vi "DriverStationSendData.vi"   [LabVIEW 2020]
doc: "This VI continously sends data from the robot to the FRC 4265 Dashboard, the joysticks, and the FIRST Driver Station. Data are only sent to the network tables when values change. Detailed sensor data are only sent when the user is currently viewing the Tune tab on the FRC 4265 Dashboard."
uses:
  GlobalDriverStationData.vi
  <vilib>/Rock Robotics/Network Tables/NT Write String Array.vi
  GlobalAutonomous.vi
  GlobalPoseAndTargeting.vi
  GlobalMiscellaneous.vi
  89115614-314f-44eb-b4c5-fafba5d31cd4.vi
  d5b4d43d-cd94-4278-ad04-5030dc28ac17.vi
  9f98788f-6f1b-4a83-a100-7d872b9f460c.vi
  47e8091e-0604-4560-b6ee-932fcc40f94c.vi
  d2dc3f3f-39b5-4c17-a933-05bbedc8d5d9.vi
  36759aca-d9c6-44a3-918a-9a0e895c718f.vi
  0620df73-5841-450f-a219-dd10bb38cbc0.vi
  fb087c59-fbb1-4979-ba7d-d29f083bcd8a.vi
  5739ca73-a30d-4c92-9c50-72d6edc45fc4.vi
  811948b9-57e2-4f47-a6f6-f2932d14082f.vi
  040c557e-2b24-4d13-8fef-d98c711cf45f.vi
  5dc304d7-e71b-4cd2-8d9d-954937278b50.vi
  296afef1-bc02-48ee-92b6-09523bb21575.vi
  5ccc8aa6-325d-4660-b060-52e30b1d582a.vi
  52d993e2-6fbc-4ee4-b085-b3f80a4c3067.vi
  63edfc8b-2713-4fb9-bbf0-712b13f7ed91.vi
  c0b3d222-824d-4eea-b194-4551ccfede72.vi
  cbbdf295-aa1d-4db8-8566-cac5820e4458.vi
  26471c2c-aca7-4047-a7cd-e40da11d04c1.vi
  a2a431f6-075f-4920-bddd-4a0a2690fbc3.vi
  d5b53c9f-0752-48c4-83e9-94c6e20357af.vi
  5e95d400-1295-40c5-af46-ec5444c3a2ff.vi
  20dd8ad3-6bbc-4cac-b559-7f798e2b6680.vi
  7b6a1411-5027-49fa-871d-ec9f81e31f95.vi
  c10cd8a7-bdb7-4c92-ac5c-00af4ab7dc85.vi
  07cec073-88f4-4f05-94a3-d05e12405c4e.vi
  948ebb5e-1fee-45f5-b788-843df8d92f11.vi
  0c9c2ce5-4f8f-4d2f-a61f-dde9fdddd21a.vi
  6883bb39-9618-44d1-87fc-0a8820399f5c.vi
  <vilib>/Rock Robotics/Network Tables/NT Write String.vi
  <vilib>/Rock Robotics/Network Tables/NT Write Number.vi
  90b8ffb3-02b0-4f37-8578-c415475fcf1f.vi
  fa7611ee-6daf-4341-84ec-bae2216748b8.vi
  94826c24-d30e-4eee-b4d4-6d626a9b9fe7.vi
  ce82ba1c-dcc2-498f-8d23-146b12230de2.vi
  e617f737-58a4-4889-9924-01a8da667f92.vi
  c227876e-c49d-4561-a8c1-0ac62d9f5df0.vi
  44842b00-b9c8-4b1f-a6e0-fc22f00ef89a.vi
  a9076398-35a2-42a7-b542-3dd64d126b59.vi
  GlobalDrivebase.vi
  0776bb0e-5b58-4af6-957d-bc8a00d122f2.vi
  <vilib>/Rock Robotics/WPI/DriverStation/WPI_DriverStationAllianceInfo.ctl
  <vilib>/Rock Robotics/Network Tables/NT Write Boolean.vi
  e0f98f21-d526-4ef5-b75c-6f3c78a33603.vi
  09cab74e-98ba-4de8-92cd-b77291f0cae9.vi
  bf36f1cc-a3b1-4189-9382-aff2debcdd91.vi
  9b798e4d-9237-4864-9935-e997a6382231.vi
  d8771982-752a-4faa-9266-2bef2163cf3a.vi
  12ad7fc7-8c22-4204-99a5-6d293ce0fad5.vi
  26bfd72d-5ff1-456c-8357-2895bcab42df.vi
  770be32f-1451-480f-be59-c95d907125ff.vi
  <vilib>/Rock Robotics/Network Tables/NT Write Float Array.vi
  8b25c428-5d86-4327-8799-14b0f475aaa3.vi
types:
  T1 = typedef "WPI_DriverStationAllianceInfo.ctl" = enum16{"Red", "Blue", "Invalid"}
  T2 = enum16{"Low Gear", "High Gear", "Transiting", "Unknown", "Force Low Gear"}
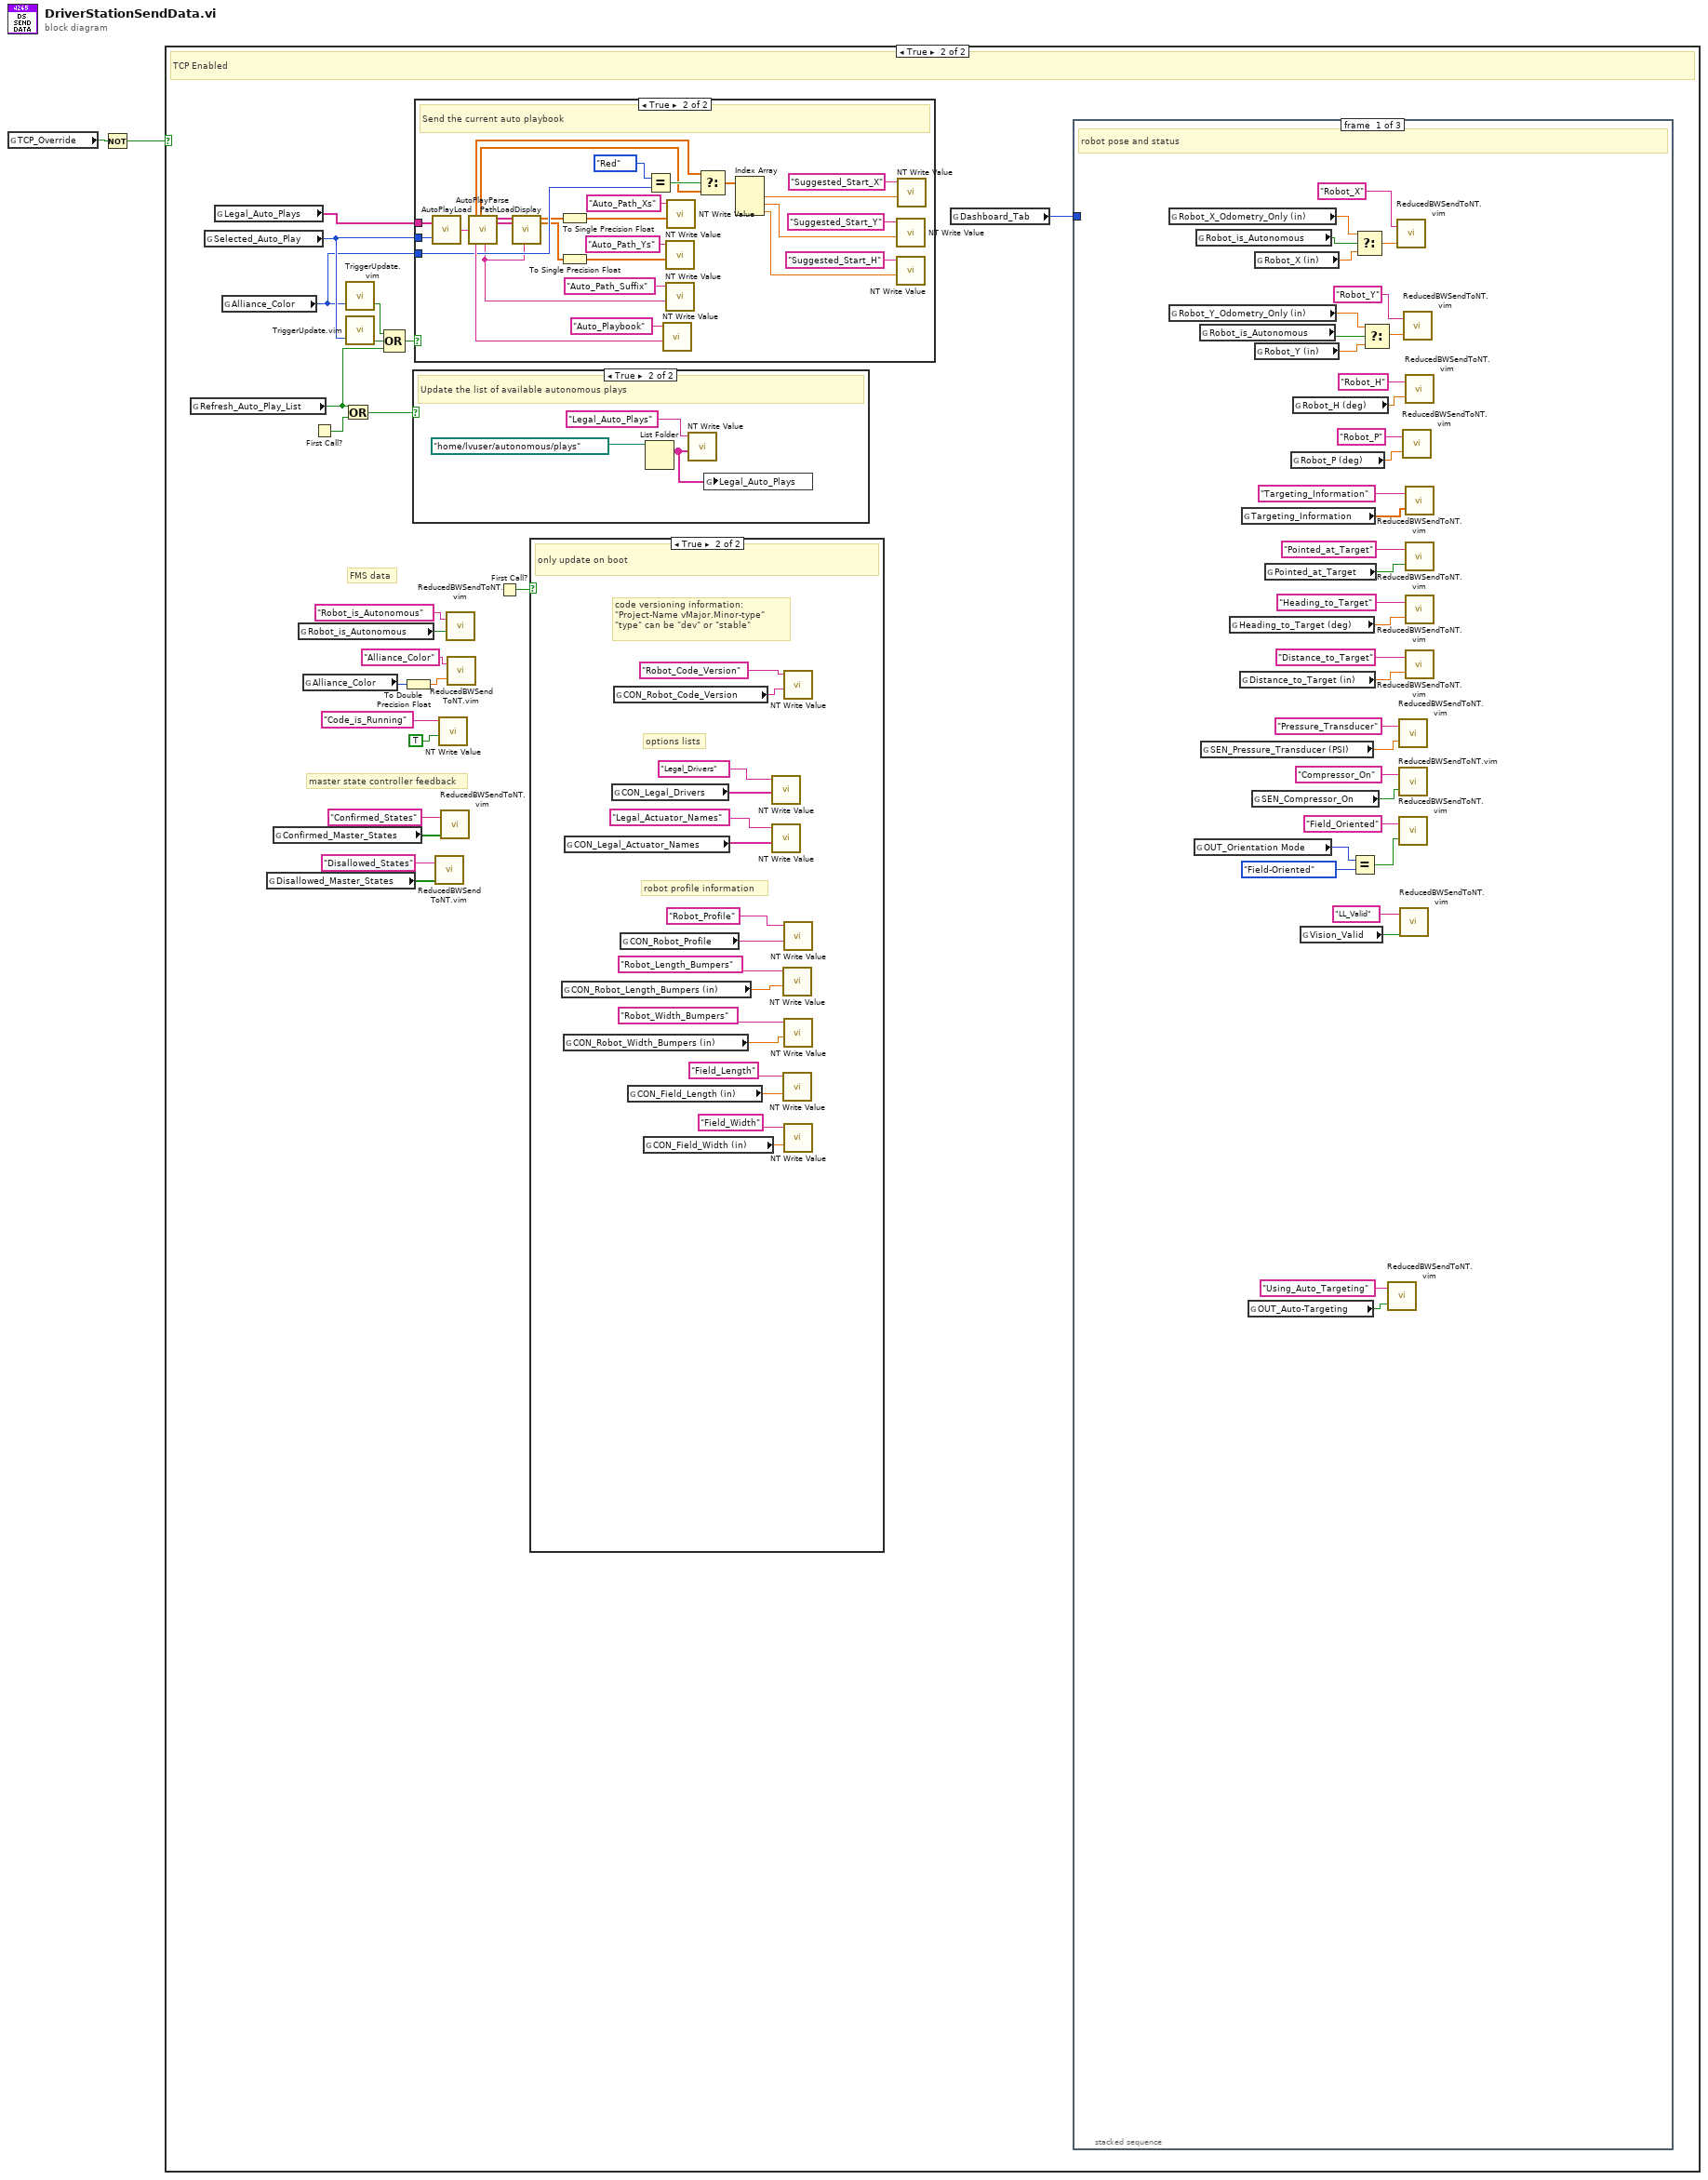
[diagram p0: block diagram]
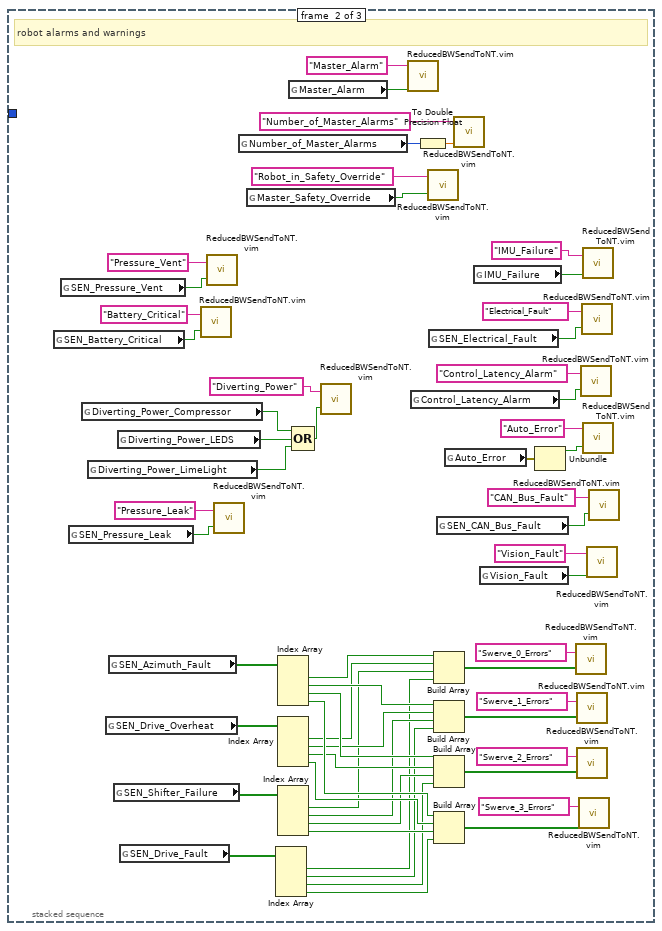
[diagram p3: hidden frame]
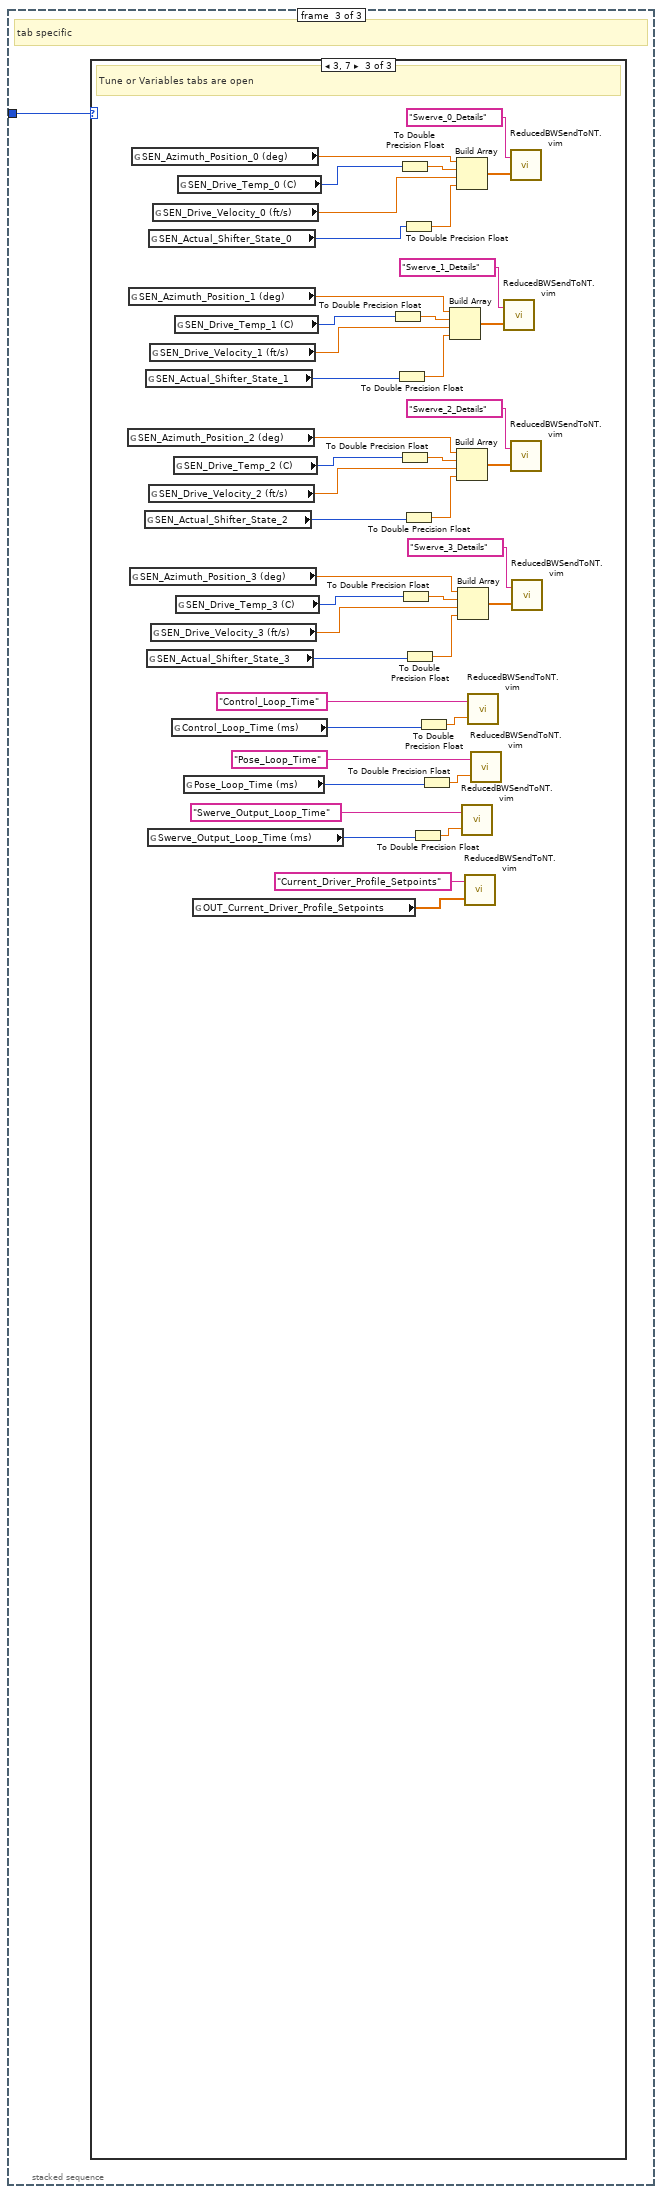
[diagram p4: hidden frame]
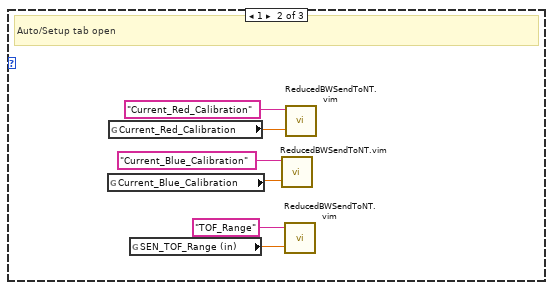
[diagram p6: hidden frame]
diagram:
  n1 = global read "GlobalDriverStationData.vi" "TCP_Override"() -> (w2:bool)
  n2 = Not(x=w2) -> (.not. x?=w1:bool)
  n3 = case shown="True" w1 {
    frame False {
      # "TCP Disabled"
    }
    frame True {
      # "FMS data"
      # "master state controller feedback"
      # "TCP Enabled"
      n4 = global read "GlobalDriverStationData.vi" "Refresh_Auto_Play_List"() -> (w20:bool)
      n5 = global read "GlobalDriverStationData.vi" "Selected_Auto_Play"() -> (w7:u16)
      n6 = global read "GlobalAutonomous.vi" "Legal_Auto_Plays"() -> (w8:string[])
      n7 = global read "GlobalDriverStationData.vi" "Alliance_Color"() -> (w5:T1)
      n8 = global read "GlobalMiscellaneous.vi" "Disallowed_Master_States"() -> (w10:bool[])
      n9 = global read "GlobalMiscellaneous.vi" "Confirmed_Master_States"() -> (w12:bool[])
      n10 = global read "GlobalDriverStationData.vi" "Robot_is_Autonomous"() -> (w16:bool)
      n11 = global read "GlobalDriverStationData.vi" "Alliance_Color"() -> (w18:T1)
      n12 = First Call?() -> (First Call?: T/F=w24:bool)
      n13 = Or(x=w20, y=w24) -> (x .or. y?=w23:bool)
      n14 = call "TriggerUpdate.vim"("Trigger"=w5) -> ("Update"=w6:bool)  [unwired: 2 in]
      n15 = call "TriggerUpdate.vim"("Trigger"=w7) -> ("Update"=w22:bool)  [unwired: 2 in]
      n16 = Compound Arithmetic op=OR(w6, w22, w20) -> (w21:bool)
      n17 = To Double Precision Float(number=w18) -> (double precision float=w14:dbl)
      n18 = case shown="True" w23 {
        frame False {
        }
        frame True {
          # "Update the list of available autonomous plays"
          n19 = List Folder(path=path "/home/lvuser/autonomous/plays") -> (filenames=w211:string[])  [unwired: 3 in, 3 out]
          n20 = call-poly <vilib>:"NT Write Value.vi"("value"=w211, "name"="Legal_Auto_Plays" ("Name")) -> ()  [unwired: 9 in, 1 out]
          n21 = global write "GlobalAutonomous.vi" "Legal_Auto_Plays"(w211) -> ()
        }
      }
      n22 = case shown="True" w21 {
        tunnel: w7 -> [_ w208]
        tunnel: w8 -> [_ w207]
        tunnel: w5 -> [_ w203]
        frame False {
        }
        frame True {
          # "Send the current auto playbook"
          n23 = call "AutoPlayLoad.vi"("Selected Auto Play"=w208, "Available Auto Plays"=w207) -> ("Loaded Auto Play"=w209:string)
          n24 = call "AutoPlayParse.vi"("Loaded Auto Play"=w209) -> ("Suggested Start Red"=w201:dbl[], "Full Auto Play Text"=w206:string, "Suggested Start Blue"=w200:dbl[], "Autonomous Path Suffix"=w190:string, "Drive Command Strings"=w192:string[], "Drive Parameter Strings"=w191:string[])  [unwired: 10 in, 3 out]
          n25 = call "PathLoadDisplay.vi"("Drive Command Strings"=w192, "Drive Parameter Strings"=w191, "Autonomous Path Suffix"=w190) -> ("Path X Coordinates (in)"=w188:dbl[], "Path Y Coordinates (in)"=w186:dbl[])  [unwired: 15 in]
          n26 = To Single Precision Float(number=w188) -> (single precision float=w185:sgl[])
          n27 = To Single Precision Float(number=w186) -> (single precision float=w184:sgl[])
          n28 = Equal?(x=WPI_DriverStationAllianceInfo."Red", y=w203) -> (x = y?=w204:bool)
          n29 = call-poly <vilib>:"NT Write Value.vi"("value"=w206, "name"="Auto_Playbook" ("Name")) -> ()  [unwired: 9 in, 1 out]
          n30 = call-poly <vilib>:"NT Write Value.vi"("value"=w184, "name"="Auto_Path_Ys" ("Name")) -> ()  [unwired: 9 in, 1 out]
          n31 = call-poly <vilib>:"NT Write Value.vi"("value"=w190, "name"="Auto_Path_Suffix" ("Name")) -> ()  [unwired: 9 in, 1 out]
          n32 = call-poly <vilib>:"NT Write Value.vi"("value"=w185, "name"="Auto_Path_Xs" ("Name")) -> ()  [unwired: 9 in, 1 out]
          n33 = Select(t=w201, s=w204, f=w200) -> (s? t:f=w199:dbl[])
          n34 = Index Array(array=w199) -> (element #1=w195:dbl, element #2=w194:dbl, element #3=w193:dbl)  [unwired: 3 in]
          n35 = call-poly <vilib>:"NT Write Value.vi"("value"=w194, "name"="Suggested_Start_Y" ("Name")) -> ()  [unwired: 9 in, 1 out]
          n36 = call-poly <vilib>:"NT Write Value.vi"("value"=w193, "name"="Suggested_Start_H" ("Name")) -> ()  [unwired: 9 in, 1 out]
          n37 = call-poly <vilib>:"NT Write Value.vi"("value"=w195, "name"="Suggested_Start_X" ("Name")) -> ()  [unwired: 9 in, 1 out]
        }
      }
      n38 = call "ReducedBWSendToNT.vim"("Value In"=w10, "NT Name"="Disallowed_States" ("Name")) -> ()  [unwired: 1 out]
      n39 = call-poly <vilib>:"NT Write Value.vi"("value"=TRUE, "name"="Code_is_Running" ("NT Name")) -> ()  [unwired: 9 in, 1 out]
      n40 = call "ReducedBWSendToNT.vim"("Value In"=w12, "NT Name"="Confirmed_States" ("Name")) -> ()  [unwired: 1 out]
      n41 = call "ReducedBWSendToNT.vim"("Value In"=w16, "NT Name"="Robot_is_Autonomous") -> ()  [unwired: 1 out]
      n42 = call "ReducedBWSendToNT.vim"("Value In"=w14, "NT Name"="Alliance_Color") -> ()  [unwired: 1 out]
      n43 = First Call?() -> (First Call?: T/F=w19:bool)
      n44 = case shown="True" w19 {
        frame False {
        }
        frame True {
          # "robot profile information"
          # "options lists"
          # "code versioning information:\n\"Project-Name vMajor.Minor-type\"\n\"type\" can be \"dev\" or \"stable\""
          # "only update on boot"
          n45 = global read "GlobalDrivebase.vi" "CON_Robot_Length_Bumpers (in)"() -> (w177:dbl)
          n46 = global read "GlobalDrivebase.vi" "CON_Robot_Width_Bumpers (in)"() -> (w176:dbl)
          n47 = global read "GlobalMiscellaneous.vi" "CON_Legal_Actuator_Names"() -> (w174:string[])
          n48 = global read "GlobalDrivebase.vi" "CON_Legal_Drivers"() -> (w175:string[])
          n49 = global read "GlobalMiscellaneous.vi" "CON_Robot_Code_Version"() -> (w172:string)
          n50 = global read "GlobalMiscellaneous.vi" "CON_Robot_Profile"() -> (w173:string)
          n51 = global read "GlobalPoseAndTargeting.vi" "CON_Field_Length (in)"() -> (w171:dbl)
          n52 = global read "GlobalPoseAndTargeting.vi" "CON_Field_Width (in)"() -> (w168:dbl)
          n53 = call-poly <vilib>:"NT Write Value.vi"("value"=w175, "name"="Legal_Drivers" ("Name")) -> ()  [unwired: 9 in, 1 out]
          n54 = call-poly <vilib>:"NT Write Value.vi"("value"=w174, "name"="Legal_Actuator_Names" ("Name")) -> ()  [unwired: 9 in, 1 out]
          n55 = call-poly <vilib>:"NT Write Value.vi"("value"=w177, "name"="Robot_Length_Bumpers" ("Name")) -> ()  [unwired: 9 in, 1 out]
          n56 = call-poly <vilib>:"NT Write Value.vi"("value"=w171, "name"="Field_Length" ("Name")) -> ()  [unwired: 9 in, 1 out]
          n57 = call-poly <vilib>:"NT Write Value.vi"("value"=w172, "name"="Robot_Code_Version" ("Name")) -> ()  [unwired: 9 in, 1 out]
          n58 = call-poly <vilib>:"NT Write Value.vi"("value"=w173, "name"="Robot_Profile" ("Name")) -> ()  [unwired: 9 in, 1 out]
          n59 = call-poly <vilib>:"NT Write Value.vi"("value"=w176, "name"="Robot_Width_Bumpers" ("Name")) -> ()  [unwired: 9 in, 1 out]
          n60 = call-poly <vilib>:"NT Write Value.vi"("value"=w168, "name"="Field_Width" ("Name")) -> ()  [unwired: 9 in, 1 out]
        }
      }
      n61 = global read "GlobalDriverStationData.vi" "Dashboard_Tab"() -> (w9:i8)
      n62 = stacked-sequence {
        tunnel: w9 -> [_ _ w118]
        frame #0 {
          # "robot pose and status"
          n63 = global read "GlobalPoseAndTargeting.vi" "Robot_X_Odometry_Only (in)"() -> (w53:dbl)
          n64 = global read "GlobalPoseAndTargeting.vi" "Robot_Y_Odometry_Only (in)"() -> (w54:dbl)
          n65 = global read "GlobalDrivebase.vi" "OUT_Orientation Mode"() -> (w37:enum16{"Robot-Oriented", "Field-Oriented"})
          n66 = global read "GlobalDriverStationData.vi" "Robot_is_Autonomous"() -> (w57:bool)
          n67 = global read "GlobalDriverStationData.vi" "Robot_is_Autonomous"() -> (w58:bool)
          n68 = global read "GlobalMiscellaneous.vi" "SEN_Pressure_Transducer (PSI)"() -> (w36:dbl)
          n69 = global read "GlobalPoseAndTargeting.vi" "Heading_to_Target (deg)"() -> (w30:dbl)
          n70 = global read "GlobalPoseAndTargeting.vi" "Distance_to_Target (in)"() -> (w28:dbl)
          n71 = global read "GlobalPoseAndTargeting.vi" "Targeting_Information"() -> (w49:dbl[])
          n72 = global read "GlobalDrivebase.vi" "OUT_Auto-Targeting"() -> (w25:bool)
          n73 = global read "GlobalMiscellaneous.vi" "SEN_Compressor_On"() -> (w35:bool)
          n74 = global read "GlobalPoseAndTargeting.vi" "Robot_X (in)"() -> (w51:dbl)
          n75 = global read "GlobalPoseAndTargeting.vi" "Robot_Y (in)"() -> (w52:dbl)
          n76 = global read "GlobalPoseAndTargeting.vi" "Pointed_at_Target"() -> (w32:bool)
          n77 = global read "GlobalPoseAndTargeting.vi" "Robot_P (deg)"() -> (w34:dbl)
          n78 = global read "GlobalPoseAndTargeting.vi" "Robot_H (deg)"() -> (w50:dbl)
          n79 = global read "GlobalPoseAndTargeting.vi" "Vision_Valid"() -> (w43:bool)
          n80 = Equal?(x=w37, y=enum16{"Robot-Oriented", "Field-Oriented"}."Field-Oriented") -> (x = y?=w44:bool)
          n81 = Select(t=w53, s=w57, f=w51) -> (s? t:f=w55:dbl)
          n82 = Select(t=w54, s=w58, f=w52) -> (s? t:f=w56:dbl)
          n83 = call "ReducedBWSendToNT.vim"("Value In"=w25, "NT Name"="Using_Auto_Targeting" ("Name")) -> ()  [unwired: 1 out]
          n84 = call "ReducedBWSendToNT.vim"("Value In"=w55, "NT Name"="Robot_X" ("Name")) -> ()  [unwired: 1 out]
          n85 = call "ReducedBWSendToNT.vim"("Value In"=w36, "NT Name"="Pressure_Transducer" ("Name")) -> ()  [unwired: 1 out]
          n86 = call "ReducedBWSendToNT.vim"("Value In"=w35, "NT Name"="Compressor_On" ("Name")) -> ()  [unwired: 1 out]
          n87 = call "ReducedBWSendToNT.vim"("Value In"=w44, "NT Name"="Field_Oriented" ("Name")) -> ()  [unwired: 1 out]
          n88 = call "ReducedBWSendToNT.vim"("Value In"=w43, "NT Name"="LL_Valid" ("Name")) -> ()  [unwired: 1 out]
          n89 = call "ReducedBWSendToNT.vim"("Value In"=w34, "NT Name"="Robot_P" ("Name")) -> ()  [unwired: 1 out]
          n90 = call "ReducedBWSendToNT.vim"("Value In"=w56, "NT Name"="Robot_Y" ("Name")) -> ()  [unwired: 1 out]
          n91 = call "ReducedBWSendToNT.vim"("Value In"=w50, "NT Name"="Robot_H" ("Name")) -> ()  [unwired: 1 out]
          n92 = call "ReducedBWSendToNT.vim"("Value In"=w49, "NT Name"="Targeting_Information" ("Name")) -> ()  [unwired: 1 out]
          n93 = call "ReducedBWSendToNT.vim"("Value In"=w32, "NT Name"="Pointed_at_Target" ("Name")) -> ()  [unwired: 1 out]
          n94 = call "ReducedBWSendToNT.vim"("Value In"=w30, "NT Name"="Heading_to_Target" ("Name")) -> ()  [unwired: 1 out]
          n95 = call "ReducedBWSendToNT.vim"("Value In"=w28, "NT Name"="Distance_to_Target" ("Name")) -> ()  [unwired: 1 out]
        }
        frame #1 {
          # "robot alarms and warnings"
          n96 = global read "GlobalMiscellaneous.vi" "SEN_Battery_Critical"() -> (w68:bool)
          n97 = global read "GlobalMiscellaneous.vi" "SEN_Pressure_Vent"() -> (w69:bool)
          n98 = global read "GlobalMiscellaneous.vi" "SEN_Pressure_Leak"() -> (w65:bool)
          n99 = global read "GlobalMiscellaneous.vi" "Diverting_Power_Compressor"() -> (w109:bool)
          n100 = global read "GlobalMiscellaneous.vi" "Diverting_Power_LimeLight"() -> (w111:bool)
          n101 = global read "GlobalDrivebase.vi" "SEN_Drive_Overheat"() -> (w71:bool[])
          n102 = global read "GlobalDrivebase.vi" "SEN_Azimuth_Fault"() -> (w72:bool[])
          n103 = global read "GlobalDrivebase.vi" "SEN_Shifter_Failure"() -> (w70:bool[])
          n104 = global read "GlobalMiscellaneous.vi" "Diverting_Power_LEDS"() -> (w110:bool)
          n105 = global read "GlobalDrivebase.vi" "SEN_Drive_Fault"() -> (w63:bool[])
          n106 = call "ReducedBWSendToNT.vim"("Value In"=w68, "NT Name"="Battery_Critical" ("Name")) -> ()  [unwired: 1 out]
          n107 = call "ReducedBWSendToNT.vim"("Value In"=w69, "NT Name"="Pressure_Vent" ("Name")) -> ()  [unwired: 1 out]
          n108 = call "ReducedBWSendToNT.vim"("Value In"=w65, "NT Name"="Pressure_Leak" ("Name")) -> ()  [unwired: 1 out]
          n109 = global read "GlobalMiscellaneous.vi" "Number_of_Master_Alarms"() -> (w116:i32)
          n110 = global read "GlobalDriverStationData.vi" "Master_Safety_Override"() -> (w112:bool)
          n111 = Index Array(array=w63) -> (element #1=w62:bool, element #2=w61:bool, element #3=w60:bool, element #4=w59:bool)  [unwired: 4 in]
          n112 = Index Array(array=w72) -> (element #1=w79:bool, element #2=w82:bool, element #3=w85:bool, element #4=w88:bool)  [unwired: 4 in]
          n113 = Index Array(array=w71) -> (element #1=w80:bool, element #2=w83:bool, element #3=w86:bool, element #4=w89:bool)  [unwired: 4 in]
          n114 = Index Array(array=w70) -> (element #1=w81:bool, element #2=w84:bool, element #3=w87:bool, element #4=w90:bool)  [unwired: 4 in]
          n115 = global read "GlobalMiscellaneous.vi" "Master_Alarm"() -> (w115:bool)
          n116 = Compound Arithmetic op=OR(w109, w110, w111) -> (w108:bool)
          n117 = call "ReducedBWSendToNT.vim"("Value In"=w108, "NT Name"="Diverting_Power" ("Name")) -> ()  [unwired: 1 out]
          n118 = call "ReducedBWSendToNT.vim"("Value In"=w115, "NT Name"="Master_Alarm" ("Name")) -> ()  [unwired: 1 out]
          n119 = global read "GlobalMiscellaneous.vi" "Control_Latency_Alarm"() -> (w66:bool)
          n120 = To Double Precision Float(number=w116) -> (double precision float=w117:dbl)
          n121 = call "ReducedBWSendToNT.vim"("Value In"=w112, "NT Name"="Robot_in_Safety_Override" ("Name")) -> ()  [unwired: 1 out]
          n122 = global read "GlobalMiscellaneous.vi" "SEN_Electrical_Fault"() -> (w67:bool)
          n123 = Build Array(w79, w80, w81, w62) -> (w91:bool[])
          n124 = Build Array(w82, w83, w84, w61) -> (w92:bool[])
          n125 = Build Array(w85, w86, w87, w60) -> (w93:bool[])
          n126 = Build Array(w88, w89, w90, w59) -> (w94:bool[])
          n127 = global read "GlobalMiscellaneous.vi" "SEN_CAN_Bus_Fault"() -> (w64:bool)
          n128 = global read "GlobalAutonomous.vi" "Auto_Error"() -> (w105:errorcluster)
          n129 = call "ReducedBWSendToNT.vim"("Value In"=w117, "NT Name"="Number_of_Master_Alarms" ("Name")) -> ()  [unwired: 1 out]
          n130 = global read "GlobalPoseAndTargeting.vi" "IMU_Failure"() -> (w107:bool)
          n131 = global read "GlobalPoseAndTargeting.vi" "Vision_Fault"() -> (w95:bool)
          n132 = Unbundle(w105) -> ("status"=w106:bool)  [unwired: 2 out]
          n133 = call "ReducedBWSendToNT.vim"("Value In"=w91, "NT Name"="Swerve_0_Errors") -> ()  [unwired: 1 out]
          n134 = call "ReducedBWSendToNT.vim"("Value In"=w92, "NT Name"="Swerve_1_Errors") -> ()  [unwired: 1 out]
          n135 = call "ReducedBWSendToNT.vim"("Value In"=w93, "NT Name"="Swerve_2_Errors") -> ()  [unwired: 1 out]
          n136 = call "ReducedBWSendToNT.vim"("Value In"=w94, "NT Name"="Swerve_3_Errors") -> ()  [unwired: 1 out]
          n137 = call "ReducedBWSendToNT.vim"("Value In"=w66, "NT Name"="Control_Latency_Alarm" ("Name")) -> ()  [unwired: 1 out]
          n138 = call "ReducedBWSendToNT.vim"("Value In"=w67, "NT Name"="Electrical_Fault" ("Name")) -> ()  [unwired: 1 out]
          n139 = call "ReducedBWSendToNT.vim"("Value In"=w107, "NT Name"="IMU_Failure" ("Name")) -> ()  [unwired: 1 out]
          n140 = call "ReducedBWSendToNT.vim"("Value In"=w106, "NT Name"="Auto_Error" ("Name")) -> ()  [unwired: 1 out]
          n141 = call "ReducedBWSendToNT.vim"("Value In"=w95, "NT Name"="Vision_Fault" ("Name")) -> ()  [unwired: 1 out]
          n142 = call "ReducedBWSendToNT.vim"("Value In"=w64, "NT Name"="CAN_Bus_Fault" ("Name")) -> ()  [unwired: 1 out]
        }
        frame #2 {
          # "tab specific"
          n143 = case shown="3, 7" w118 {
            frame 0, Default {
              # "no tab open"
            }
            frame 1 {
              # "Auto/Setup tab open"
              n144 = global read "GlobalPoseAndTargeting.vi" "Current_Blue_Calibration"() -> (w121:dbl)
              n145 = global read "GlobalPoseAndTargeting.vi" "Current_Red_Calibration"() -> (w124:dbl)
              n146 = global read "GlobalMiscellaneous.vi" "SEN_TOF_Range (in)"() -> (w120:dbl)
              n147 = call "ReducedBWSendToNT.vim"("Value In"=w121, "NT Name"="Current_Blue_Calibration") -> ()  [unwired: 1 out]
              n148 = call "ReducedBWSendToNT.vim"("Value In"=w120, "NT Name"="TOF_Range") -> ()  [unwired: 1 out]
              n149 = call "ReducedBWSendToNT.vim"("Value In"=w124, "NT Name"="Current_Red_Calibration") -> ()  [unwired: 1 out]
            }
            frame 3, 7 {
              # "Tune or Variables tabs are open"
              n150 = global read "GlobalDrivebase.vi" "SEN_Azimuth_Position_2 (deg)"() -> (w137:dbl)
              n151 = global read "GlobalDrivebase.vi" "SEN_Azimuth_Position_1 (deg)"() -> (w141:dbl)
              n152 = global read "GlobalDrivebase.vi" "SEN_Azimuth_Position_3 (deg)"() -> (w133:dbl)
              n153 = global read "GlobalDrivebase.vi" "SEN_Azimuth_Position_0 (deg)"() -> (w145:dbl)
              n154 = global read "GlobalDrivebase.vi" "SEN_Actual_Shifter_State_2"() -> (w134:T2)
              n155 = global read "GlobalDrivebase.vi" "SEN_Actual_Shifter_State_1"() -> (w138:T2)
              n156 = global read "GlobalDrivebase.vi" "SEN_Actual_Shifter_State_3"() -> (w130:T2)
              n157 = global read "GlobalMiscellaneous.vi" "Swerve_Output_Loop_Time (ms)"() -> (w125:u32)
              n158 = global read "GlobalDrivebase.vi" "SEN_Actual_Shifter_State_0"() -> (w142:T2)
              n159 = global read "GlobalDrivebase.vi" "SEN_Drive_Velocity_2 (ft/s)"() -> (w135:dbl)
              n160 = global read "GlobalDrivebase.vi" "SEN_Drive_Velocity_1 (ft/s)"() -> (w139:dbl)
              n161 = global read "GlobalDrivebase.vi" "SEN_Drive_Velocity_3 (ft/s)"() -> (w131:dbl)
              n162 = global read "GlobalDrivebase.vi" "SEN_Drive_Velocity_0 (ft/s)"() -> (w143:dbl)
              n163 = global read "GlobalMiscellaneous.vi" "Control_Loop_Time (ms)"() -> (w129:u32)
              n164 = global read "GlobalDrivebase.vi" "SEN_Drive_Temp_2 (C)"() -> (w136:u8)
              n165 = global read "GlobalDrivebase.vi" "SEN_Drive_Temp_1 (C)"() -> (w140:u8)
              n166 = global read "GlobalDrivebase.vi" "SEN_Drive_Temp_3 (C)"() -> (w132:u8)
              n167 = global read "GlobalDrivebase.vi" "SEN_Drive_Temp_0 (C)"() -> (w144:u8)
              n168 = global read "GlobalMiscellaneous.vi" "Pose_Loop_Time (ms)"() -> (w128:u32)
              n169 = global read "GlobalDrivebase.vi" "OUT_Current_Driver_Profile_Setpoints"() -> (w146:dbl[])
              n170 = To Double Precision Float(number=w140) -> (double precision float=w158:dbl)
              n171 = To Double Precision Float(number=w138) -> (double precision float=w157:dbl)
              n172 = To Double Precision Float(number=w144) -> (double precision float=w162:dbl)
              n173 = To Double Precision Float(number=w136) -> (double precision float=w154:dbl)
              n174 = To Double Precision Float(number=w132) -> (double precision float=w150:dbl)
              n175 = To Double Precision Float(number=w142) -> (double precision float=w161:dbl)
              n176 = To Double Precision Float(number=w134) -> (double precision float=w153:dbl)
              n177 = To Double Precision Float(number=w130) -> (double precision float=w149:dbl)
              n178 = To Double Precision Float(number=w125) -> (double precision float=w126:dbl)
              n179 = To Double Precision Float(number=w129) -> (double precision float=w166:dbl)
              n180 = To Double Precision Float(number=w128) -> (double precision float=w164:dbl)
              n181 = Build Array(w141, w158, w139, w157) -> (w156:dbl[])
              n182 = Build Array(w145, w162, w143, w161) -> (w160:dbl[])
              n183 = Build Array(w137, w154, w135, w153) -> (w152:dbl[])
              n184 = Build Array(w133, w150, w131, w149) -> (w148:dbl[])
              n185 = call "ReducedBWSendToNT.vim"("Value In"=w126, "NT Name"="Swerve_Output_Loop_Time" ("Name")) -> ()  [unwired: 1 out]
              n186 = call "ReducedBWSendToNT.vim"("Value In"=w146, "NT Name"="Current_Driver_Profile_Setpoints" ("Name")) -> ()  [unwired: 1 out]
              n187 = call "ReducedBWSendToNT.vim"("Value In"=w166, "NT Name"="Control_Loop_Time" ("Name")) -> ()  [unwired: 1 out]
              n188 = call "ReducedBWSendToNT.vim"("Value In"=w164, "NT Name"="Pose_Loop_Time" ("Name")) -> ()  [unwired: 1 out]
              n189 = call "ReducedBWSendToNT.vim"("Value In"=w156, "NT Name"="Swerve_1_Details") -> ()  [unwired: 1 out]
              n190 = call "ReducedBWSendToNT.vim"("Value In"=w160, "NT Name"="Swerve_0_Details") -> ()  [unwired: 1 out]
              n191 = call "ReducedBWSendToNT.vim"("Value In"=w152, "NT Name"="Swerve_2_Details") -> ()  [unwired: 1 out]
              n192 = call "ReducedBWSendToNT.vim"("Value In"=w148, "NT Name"="Swerve_3_Details") -> ()  [unwired: 1 out]
            }
          }
        }
      }
    }
  }
